vi "array_resize_test.vi"(1 "Value 3":cluster{"MSG":i16, "Param":i32, "type":i16}[](array[cluster]), 2 "Arr Refnum":refnum<vi>) -> ()   [LabVIEW 2010]
uses:
  VB.dll
panel:
  out "arg1":cluster{"MSG":i16, "Param":i32, "type":i16}[](array[cluster])
  in  "Cluster":cluster{"MSG":i16, "Param":i32, "type":i16}
  in  "algOutputMsgs":cluster{"MSG":i16, "Param":i32, "type":i16}[](array[cluster])
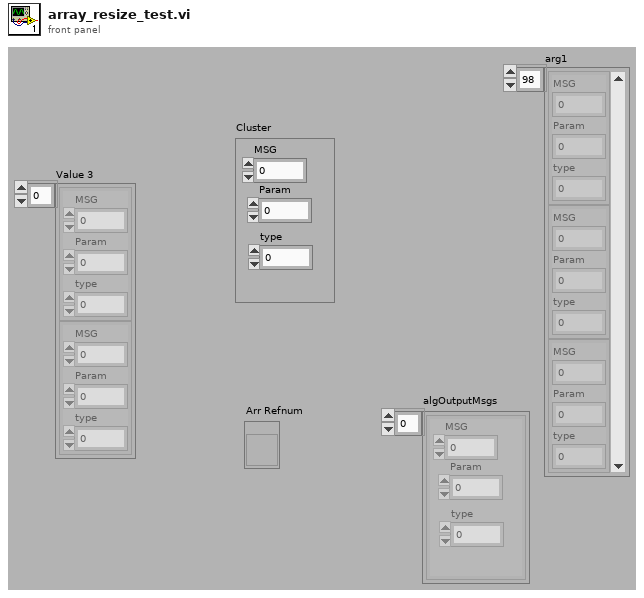
[diagram p1: front panel]
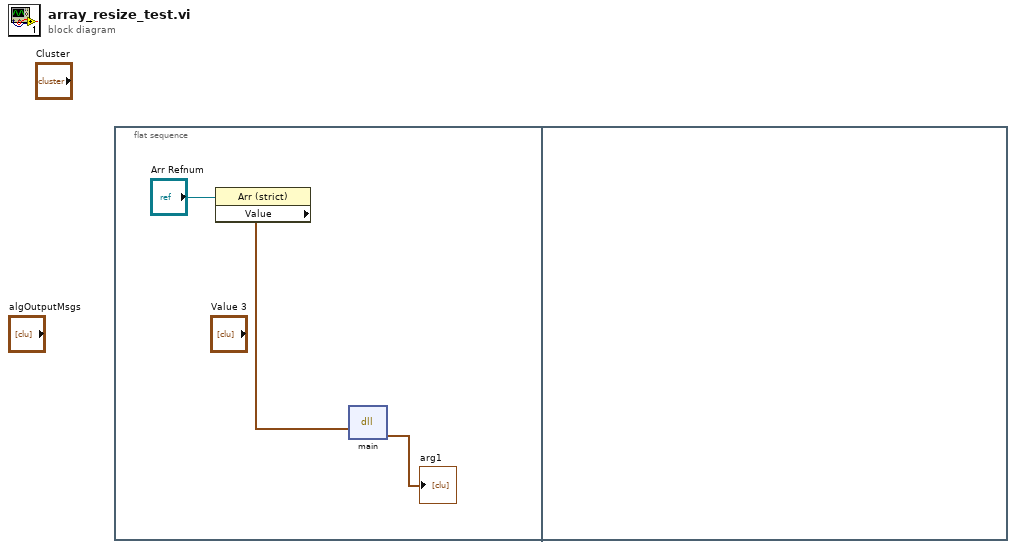
[diagram p0: block diagram]
diagram:
  n1 = flat-sequence {
    frame #0 {
      n2 = property class="Arr (strict)"(reference="Arr Refnum") -> ("Value"=w2:cluster{"MSG":i16, "Param":i32, "type":i16}[])  [unwired: 1 in, 2 out]
      n3 = dll-call lib="D:/VB.dll" fn="main"("arg1"=w2) -> ("arg1"=→"arg1":cluster{"MSG":i16, "Param":i32, "type":i16}[])  [unwired: 4 in, 2 out]
    }
    frame #1 {
    }
  }
